vi "Measure-Power_PM16-121.vi"(8 "error in (no error)":errorcluster {"code" format="%.0x"}, 11 "instrument handle":refnum<visa-resource-name>) -> (0 "error out":errorcluster, 2 "Power":dbl, 3 "instrument handle out":refnum<visa-resource-name>)   [LabVIEW 2018]
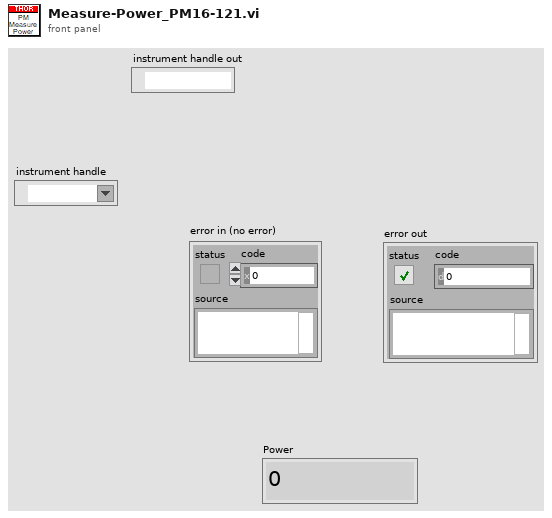
[diagram p1: front panel]
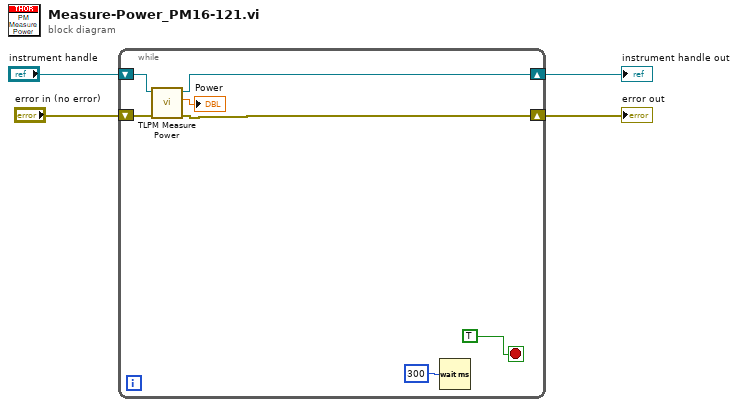
[diagram p0: block diagram]
diagram:
  n1 = while {
    shift-right: [w7] -> w1
    shift-left: "error in (no error)" -> [w9]
    shift-right: [w8] -> w2
    shift-left: "instrument handle" -> [w10]
    stop <- TRUE stop-if-true
    n2 = call "TLPM Measure Power.vi"("error in (no error)"=w9, "instrument handle"=w10) -> ("error out"=w7:errorcluster, "Power"=→"Power":dbl, "instrument handle out"=w8:refnum<visa-resource-name>)  [unwired: 7 in]
    n3 = Wait (ms)(milliseconds to wait=u32 300) -> ()  [unwired: 1 out]
  }
  "error out" <- w1
  "instrument handle out" <- w2
